vi "Velocity After Board Collision.vi"(7 "Collision in":T1, 10 "Movable in":refnum<class "Movable.lvclass">) -> (2 "Movable out":refnum<class "Movable.lvclass">)   [LabVIEW 2021, in "Game Board.lvclass"]
doc: "MIT Licence\nCopyright (c) 2024 David Grollier"
uses:
  Game Board.lvclass
  Game Board Component/Movable/Movable.lvclass
  Collision/Ball-Edge/Collision type.ctl
  Collision/Ball-Edge/Ball-Edge.lvclass
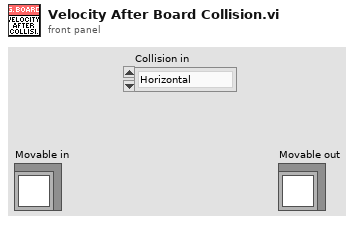
[diagram p1: front panel]
types:
  T1 = typedef "Ball-Edge.lvclass/Collision type.ctl" = enum16{"Horizontal", "Vertical", "Corner"}
  T2 = typedef "Velocity.ctl" = cluster{"Vx":dbl, "Vy":dbl}
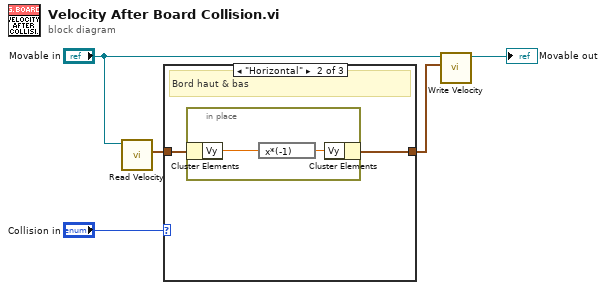
[diagram p0: block diagram]
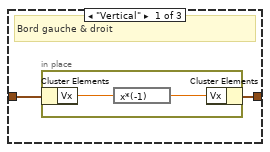
[diagram p2: hidden frame]
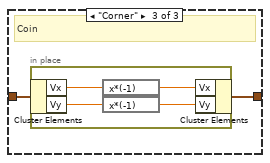
[diagram p3: hidden frame]
diagram:
  n1 = call-dynamic "Read Velocity.vi"("Movable in"="Movable in") -> ("Velocity"=w5:T2)  [unwired: 10 in]
  n2 = case shown="\"Horizontal\"" "Collision in" {
    tunnel: w5 -> [w7 w11 w15]
    tunnel: [w6 w10 w14] -> w3
    frame "Vertical" {
      # "Bord gauche & droit"
      n3 = in-place {
        n4 = in-place-cluster #1(w7) -> ("Vx"=w9:dbl)
        n5 = expression code="x*(-1)"(w9) -> (w8:dbl)
        n6 = in-place-cluster #1("Vx"=w8) -> (w6:T2)
      }
    }
    frame "Horizontal" {
      # "Bord haut & bas"
      n7 = in-place {
        n8 = in-place-cluster #2(w11) -> ("Vy"=w13:dbl)
        n9 = expression code="x*(-1)"(w13) -> (w12:dbl)
        n10 = in-place-cluster #2("Vy"=w12) -> (w10:T2)
      }
    }
    frame "Corner" {
      # "Coin"
      n11 = in-place {
        n12 = in-place-cluster #3(w15) -> ("Vx"=w17:dbl, "Vy"=w19:dbl)
        n13 = expression code="x*(-1)"(w17) -> (w16:dbl)
        n14 = expression code="x*(-1)"(w19) -> (w18:dbl)
        n15 = in-place-cluster #3("Vx"=w16, "Vy"=w18) -> (w14:T2)
      }
    }
  }
  n16 = call "Write Velocity.vi"("Velocity"=w3, "Movable in"="Movable in") -> ("Movable out"=→"Movable out":refnum<class "Movable.lvclass">)  [unwired: 9 in]
